vi "Store Load Cell Reading.vi"(8 "error in (no error)":errorcluster, 11 "Model in":refnum<class "Model.lvclass">) -> (0 "error out":errorcluster, 3 "Model out":refnum<class "Model.lvclass">)   [LabVIEW 2016, in "Model.lvclass"]
uses:
  Model.lvclass
  Model.lvclass/Model.ctl
  common_rt_hpilc/HPILC/HPILC.lvclass/HPILC.ctl
  common_rt_hpilc/HPILC/HPILC.lvclass
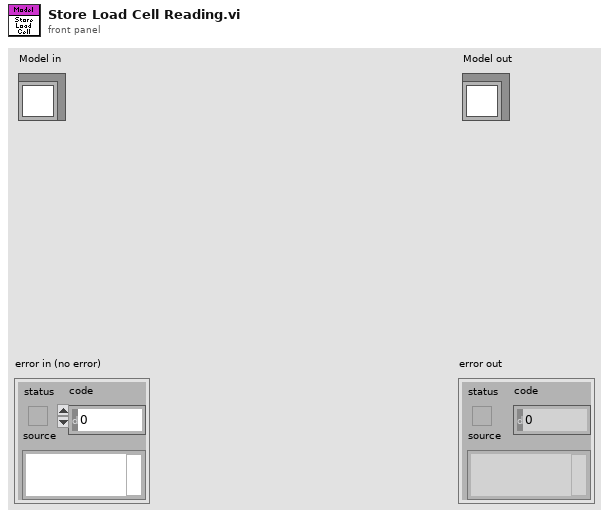
[diagram p1: front panel]
types:
  T1 = typedef "RTHPILC.lvlib/HPData.ctl" = cluster{"Constants":T2, "Command":T3, "Telemetry":T4, "Responses":T5, "Timings":T7}
  T2 = typedef "RTHPILC.lvlib/HPConstants.ctl" = cluster{"ID":i16, "ReferencePosition":i32}
  T3 = typedef "RTHPILC.lvlib/HPCommand.ctl" = cluster{"Steps":i8}
  T4 = typedef "RTHPILC.lvlib/HPTelemetry.ctl" = cluster{"ILCFault":bool, "LimitSwitchCWOperated":bool, "LimitSwitchCCWOperated":bool, "BroadcastCounter":u8, "SSIEncoderValue":i32, "LoadCellForce":sgl}
  T5 = typedef "RTHPILC.lvlib/HPResponses.ctl" = cluster{"StepMotor":T6, "ForceAndStatus":T6}
  T6 = typedef "RTModbus.lvlib/ExceptionCodes.ctl" = u16
  T7 = typedef "RTHPILC.lvlib/HPTimings.ctl" = cluster{"BroadcastStepMotor":u32, "ForceAndStatus":u32, "FreezeSensorValues":u32, "StepMotor":u32}
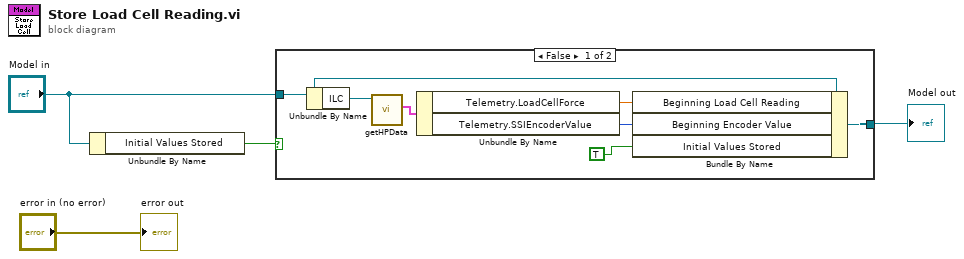
[diagram p0: block diagram]
diagram:
  n1 = Unbundle By Name("Model in") -> ("Initial Values Stored"=w1:bool)
  n2 = case shown="False" w1 {
    tunnel: [w9 w12] -> w4
    tunnel: "Model in" -> [w8 w12]
    frame False {
      n3 = Unbundle By Name(w8) -> ("ILC"=w11:refnum<class "HPILC.lvclass">)
      n4 = call "getHPData.vi"("HPILC in"=w11) -> ("HPData"=w10:T1)  [unwired: 9 in, 1 out]
      n5 = Unbundle By Name(w10) -> ("Telemetry.LoadCellForce"=w7:sgl, "Telemetry.SSIEncoderValue"=w6:i32)
      n6 = Bundle By Name(cluster=w8, "Beginning Load Cell Reading"=w7, "Beginning Encoder Value"=w6, "Initial Values Stored"=TRUE) -> (w9:refnum<class "Model.lvclass">)
    }
    frame True {
    }
  }
  "Model out" <- w4
  "error out" <- "error in (no error)"
